vi "Parse xPG Status.vi"(7 "xPG Status":string="ActiveError=0x00\r\nStimulationStateActive=NO\r\nRampingStatusActive=NO\r\nIncrementLockoutActive=NO\r\nBootloaderMode=NO\r\nP1_Selectable=YES\r\nP2_Selectable=YES\r\nP3_Selectable=YES\r\nP4_Selectable=YES\r\nP5_Selectable=YES\r\nP6_Selectable=YES\r\nP7_Selectable=YES\r\nP8_Selectable=YES\r\nP9_Selectable=YES\r\nP10_Selectable=YES\r\nSelectedProgram=0\r\nPA_Defined=NO\r\nPB_Defined=NO\r\nPC_Defined=NO\r\nPD_Defined=NO\r\nPulseVirtualAmplitudeStepIndex=0\r\nxPgBatteryState=XPG_BATT_HIGH-3\r\nChargingError=0\r\nStimState=Inactive") -> (2 "BootloaderMode":string, 3 "StimulationStateActive":string)   [LabVIEW 2010]
doc: "This function parses an xPG status string to obtain the StimulationStateActive and BootloaderMode status."
panel:
  in  "BootloaderMode Key":string="BootloaderMode="
  in  "StimulationStateActive Key":string="StimulationStateActive="
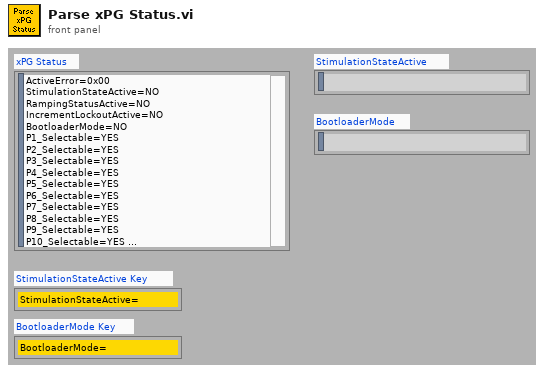
[diagram p1: front panel]
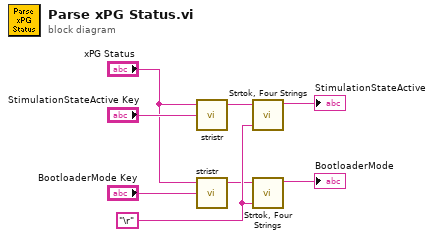
[diagram p0: block diagram]
diagram:
  w6 = "\r" ("delimiters (\\s\\t\\r\\n=)")
  n1 = call "stristr.vi"("Substring"="StimulationStateActive Key", "Input String"="xPG Status") -> ("match + rest of string"=w5:string)  [unwired: 1 in, 2 out]
  n2 = call "stristr.vi"("Substring"="BootloaderMode Key", "Input String"="xPG Status") -> ("match + rest of string"=w2:string)  [unwired: 1 in, 2 out]
  n3 = call "Strtok, Four Strings.vi"("delimiters (\\s\\t\\r\\n=)"=w6, "input string"=w5) -> ("token 1"=→"StimulationStateActive":string)  [unwired: 1 in, 3 out]
  n4 = call "Strtok, Four Strings.vi"("delimiters (\\s\\t\\r\\n=)"=w6, "input string"=w2) -> ("token 1"=→"BootloaderMode":string)  [unwired: 1 in, 3 out]
